vi "Scrap.vi"() -> ()   [LabVIEW 2023]
uses:
  <vilib>/addons/database/Connection.llb/DB Tools Open Connec (String).vi
  <vilib>/regexp/Match Regular Expression.xnode
  <vilib>/addons/database/NI_Database_API.lvlib
panel:
  in  "Quantity":dbl=1.0 min=1.0 max=20.0 step=1.0
  out "DC_SN":string
  in  "Error Code (Electrical)":string(combo)="C30 - Activity Dip"
  in  "Error Code (Electrical +)":string(combo)="C37 - G-Sensitivity"
  in  "Error Code (Post Testing)":string(combo)="C40 - Tinning"
  in  "Work Order":string
  in  "DC_SN":string
  in  "Employee Number":string
  in  "Enter":bool
  in  "Exit":bool
  in  "Comment":string
  in  "Error Code (Pre-Clean Room)":string(combo)="C14 - Dropped"
  in  "Error Code (Post Clean Room)":string(combo)="C38 - Short"
  in  "Location":string(combo)
  in  "Error Code (Clean Room)":string(combo)="C16 - No Oscillate"
  # "Scrapping"
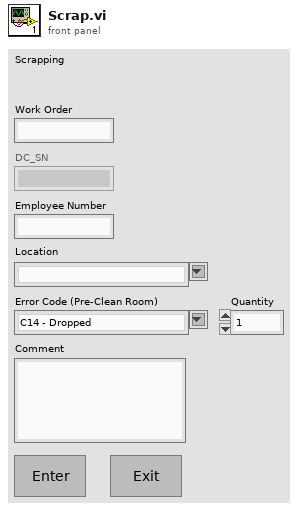
[diagram p1: front panel]
types:
  T1 = typedef "NI_Database_API.lvlib/Conn ObjectReference.ctl" = refnum<k1>
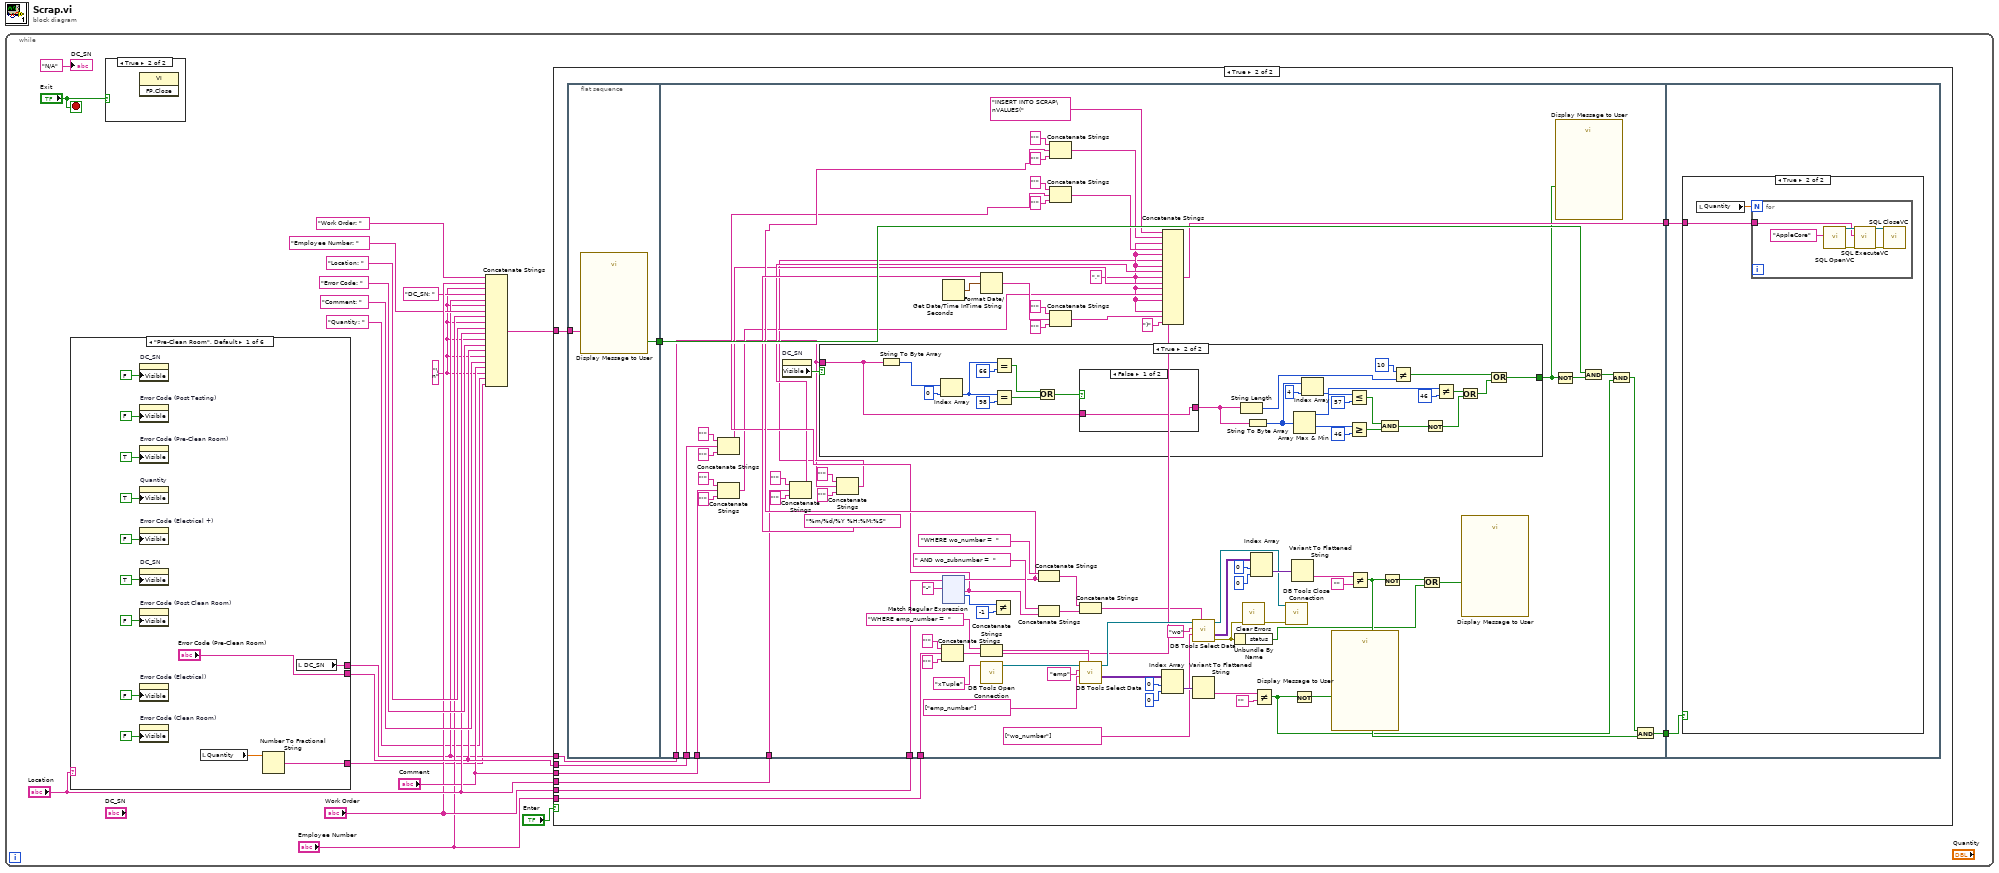
[diagram p0: block diagram]
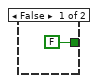
[diagram p4: hidden frame]
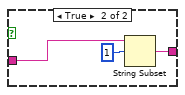
[diagram p5: hidden frame]
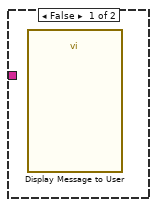
[diagram p6: hidden frame]
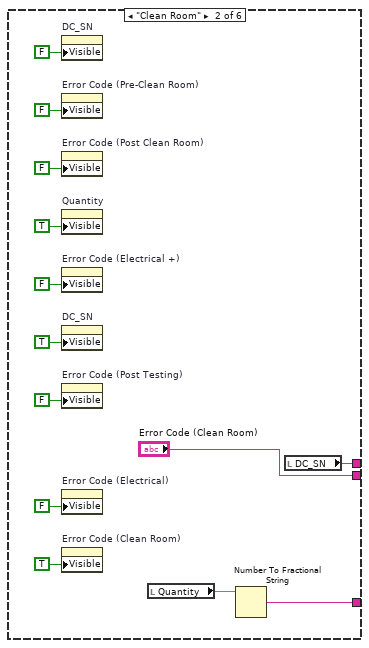
[diagram p7: hidden frame]
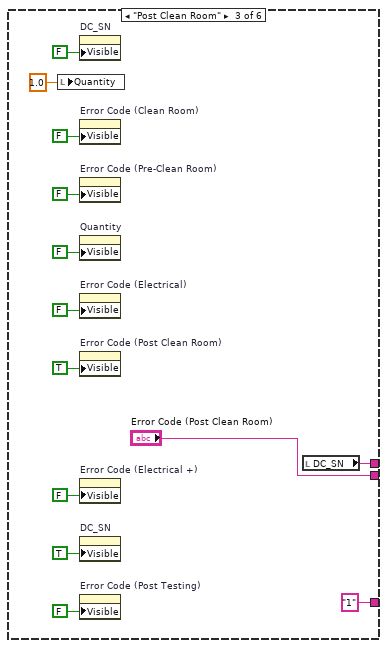
[diagram p8: hidden frame]
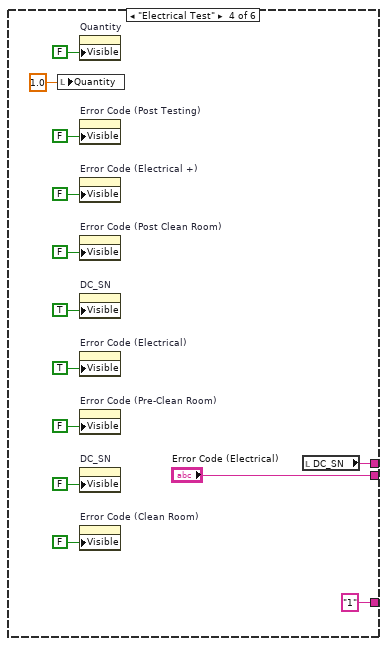
[diagram p9: hidden frame]
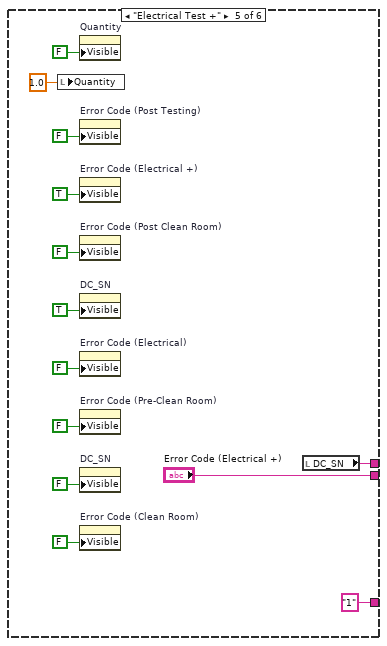
[diagram p10: hidden frame]
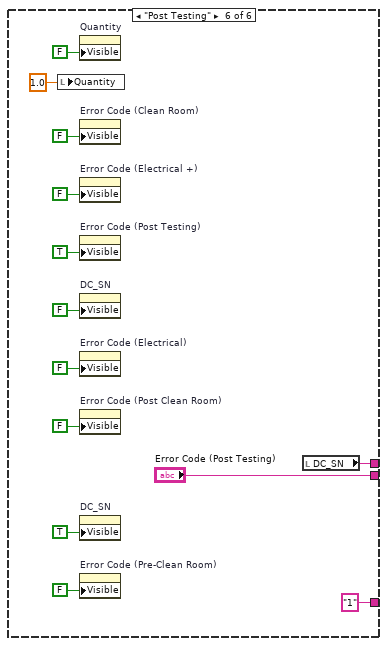
[diagram p11: hidden frame]
diagram:
  n1 = while {
    stop <- "Exit" stop-if-true
    w3 = "\n" ("string")
    n2 = case shown="\"Pre-Clean Room\", Default" "Location" {
      tunnel: ["Error Code (Pre-Clean Room)" "Error Code (Clean Room)" "Error Code (Post Clean Room)" "Error Code (Electrical)" "Error Code (Electrical +)" "Error Code (Post Testing)"] -> w13
      tunnel: [w279 w292 w305 w320 w333 w344] -> w6
      tunnel: [w276 w289 "1" "1" "1" "1"] -> w1
      frame "Pre-Clean Room", Default {
        n3 = property on="DC_SN" class="Str"("Visible"=FALSE) -> ()  [unwired: 2 in, 2 out]
        n4 = property on="Error Code (Post Testing)" class="CmbBox"("Visible"=FALSE) -> ()  [unwired: 2 in, 2 out]
        n5 = property on="Error Code (Pre-Clean Room)" class="CmbBox"("Visible"=TRUE) -> ()  [unwired: 2 in, 2 out]
        n6 = property on="Quantity" class="DigNum (strict)"("Visible"=TRUE) -> ()  [unwired: 2 in, 2 out]
        n7 = property on="Error Code (Electrical +)" class="CmbBox"("Visible"=FALSE) -> ()  [unwired: 2 in, 2 out]
        n8 = property on="DC_SN" class="Str"("Visible"=TRUE) -> ()  [unwired: 2 in, 2 out]
        n9 = property on="Error Code (Post Clean Room)" class="CmbBox"("Visible"=FALSE) -> ()  [unwired: 2 in, 2 out]
        n10 = property on="Error Code (Electrical)" class="CmbBox"("Visible"=FALSE) -> ()  [unwired: 2 in, 2 out]
        n11 = property on="Error Code (Clean Room)" class="CmbBox"("Visible"=FALSE) -> ()  [unwired: 2 in, 2 out]
        n12 = local read "Quantity"() -> (w277:dbl)
        n13 = Number To Fractional String(number=w277) -> (F-format string=w276:string)  [unwired: 3 in]
        n14 = local read "DC_SN"() -> (w279:string)
      }
      frame "Clean Room" {
        n15 = property on="DC_SN" class="Str"("Visible"=FALSE) -> ()  [unwired: 2 in, 2 out]
        n16 = property on="Error Code (Pre-Clean Room)" class="CmbBox"("Visible"=FALSE) -> ()  [unwired: 2 in, 2 out]
        n17 = property on="Error Code (Post Clean Room)" class="CmbBox"("Visible"=FALSE) -> ()  [unwired: 2 in, 2 out]
        n18 = property on="Quantity" class="DigNum (strict)"("Visible"=TRUE) -> ()  [unwired: 2 in, 2 out]
        n19 = property on="Error Code (Electrical +)" class="CmbBox"("Visible"=FALSE) -> ()  [unwired: 2 in, 2 out]
        n20 = property on="DC_SN" class="Str"("Visible"=TRUE) -> ()  [unwired: 2 in, 2 out]
        n21 = property on="Error Code (Post Testing)" class="CmbBox"("Visible"=FALSE) -> ()  [unwired: 2 in, 2 out]
        n22 = property on="Error Code (Electrical)" class="CmbBox"("Visible"=FALSE) -> ()  [unwired: 2 in, 2 out]
        n23 = property on="Error Code (Clean Room)" class="CmbBox"("Visible"=TRUE) -> ()  [unwired: 2 in, 2 out]
        n24 = local read "Quantity"() -> (w290:dbl)
        n25 = Number To Fractional String(number=w290) -> (F-format string=w289:string)  [unwired: 3 in]
        n26 = local read "DC_SN"() -> (w292:string)
      }
      frame "Post Clean Room" {
        n27 = local write "Quantity"(1.0 ("Quantity")) -> ()
        n28 = property on="DC_SN" class="Str"("Visible"=FALSE) -> ()  [unwired: 2 in, 2 out]
        n29 = property on="Error Code (Clean Room)" class="CmbBox"("Visible"=FALSE) -> ()  [unwired: 2 in, 2 out]
        n30 = property on="Error Code (Pre-Clean Room)" class="CmbBox"("Visible"=FALSE) -> ()  [unwired: 2 in, 2 out]
        n31 = property on="Quantity" class="DigNum (strict)"("Visible"=FALSE) -> ()  [unwired: 2 in, 2 out]
        n32 = property on="Error Code (Electrical)" class="CmbBox"("Visible"=FALSE) -> ()  [unwired: 2 in, 2 out]
        n33 = property on="Error Code (Post Clean Room)" class="CmbBox"("Visible"=TRUE) -> ()  [unwired: 2 in, 2 out]
        n34 = property on="Error Code (Electrical +)" class="CmbBox"("Visible"=FALSE) -> ()  [unwired: 2 in, 2 out]
        n35 = property on="DC_SN" class="Str"("Visible"=TRUE) -> ()  [unwired: 2 in, 2 out]
        n36 = property on="Error Code (Post Testing)" class="CmbBox"("Visible"=FALSE) -> ()  [unwired: 2 in, 2 out]
        n37 = local read "DC_SN"() -> (w305:string)
      }
      frame "Electrical Test" {
        n38 = local write "Quantity"(1.0 ("Quantity")) -> ()
        n39 = property on="Quantity" class="DigNum (strict)"("Visible"=FALSE) -> ()  [unwired: 2 in, 2 out]
        n40 = property on="Error Code (Post Testing)" class="CmbBox"("Visible"=FALSE) -> ()  [unwired: 2 in, 2 out]
        n41 = property on="Error Code (Electrical +)" class="CmbBox"("Visible"=FALSE) -> ()  [unwired: 2 in, 2 out]
        n42 = property on="Error Code (Post Clean Room)" class="CmbBox"("Visible"=FALSE) -> ()  [unwired: 2 in, 2 out]
        n43 = property on="DC_SN" class="Str"("Visible"=TRUE) -> ()  [unwired: 2 in, 2 out]
        n44 = property on="Error Code (Electrical)" class="CmbBox"("Visible"=TRUE) -> ()  [unwired: 2 in, 2 out]
        n45 = property on="Error Code (Pre-Clean Room)" class="CmbBox"("Visible"=FALSE) -> ()  [unwired: 2 in, 2 out]
        n46 = property on="DC_SN" class="Str"("Visible"=FALSE) -> ()  [unwired: 2 in, 2 out]
        n47 = property on="Error Code (Clean Room)" class="CmbBox"("Visible"=FALSE) -> ()  [unwired: 2 in, 2 out]
        n48 = local read "DC_SN"() -> (w320:string)
      }
      frame "Electrical Test +" {
        n49 = local write "Quantity"(1.0 ("Quantity")) -> ()
        n50 = property on="Quantity" class="DigNum (strict)"("Visible"=FALSE) -> ()  [unwired: 2 in, 2 out]
        n51 = property on="Error Code (Post Testing)" class="CmbBox"("Visible"=FALSE) -> ()  [unwired: 2 in, 2 out]
        n52 = property on="Error Code (Electrical +)" class="CmbBox"("Visible"=TRUE) -> ()  [unwired: 2 in, 2 out]
        n53 = property on="Error Code (Post Clean Room)" class="CmbBox"("Visible"=FALSE) -> ()  [unwired: 2 in, 2 out]
        n54 = property on="DC_SN" class="Str"("Visible"=TRUE) -> ()  [unwired: 2 in, 2 out]
        n55 = property on="Error Code (Electrical)" class="CmbBox"("Visible"=FALSE) -> ()  [unwired: 2 in, 2 out]
        n56 = property on="Error Code (Pre-Clean Room)" class="CmbBox"("Visible"=FALSE) -> ()  [unwired: 2 in, 2 out]
        n57 = property on="DC_SN" class="Str"("Visible"=FALSE) -> ()  [unwired: 2 in, 2 out]
        n58 = property on="Error Code (Clean Room)" class="CmbBox"("Visible"=FALSE) -> ()  [unwired: 2 in, 2 out]
        n59 = local read "DC_SN"() -> (w333:string)
      }
      frame "Post Testing" {
        n60 = local write "Quantity"(1.0 ("Quantity")) -> ()
        n61 = property on="Quantity" class="DigNum (strict)"("Visible"=FALSE) -> ()  [unwired: 2 in, 2 out]
        n62 = property on="Error Code (Clean Room)" class="CmbBox"("Visible"=FALSE) -> ()  [unwired: 2 in, 2 out]
        n63 = property on="Error Code (Electrical +)" class="CmbBox"("Visible"=FALSE) -> ()  [unwired: 2 in, 2 out]
        n64 = property on="Error Code (Post Testing)" class="CmbBox"("Visible"=TRUE) -> ()  [unwired: 2 in, 2 out]
        n65 = property on="DC_SN" class="Str"("Visible"=FALSE) -> ()  [unwired: 2 in, 2 out]
        n66 = property on="Error Code (Electrical)" class="CmbBox"("Visible"=FALSE) -> ()  [unwired: 2 in, 2 out]
        n67 = property on="Error Code (Post Clean Room)" class="CmbBox"("Visible"=FALSE) -> ()  [unwired: 2 in, 2 out]
        n68 = property on="DC_SN" class="Str"("Visible"=TRUE) -> ()  [unwired: 2 in, 2 out]
        n69 = property on="Error Code (Pre-Clean Room)" class="CmbBox"("Visible"=FALSE) -> ()  [unwired: 2 in, 2 out]
        n70 = local read "DC_SN"() -> (w344:string)
      }
    }
    n71 = case shown="True" "Exit" {
      frame False {
      }
      frame True {
        n72 = invoke class="VI" method="FP.Close"() -> ()  [unwired: 3 in, 3 out]
      }
    }
    n73 = Concatenate Strings("Work Order: " ("string"), "Work Order", w3, "DC_SN: " ("string"), w6, w3, "Employee Number: " ("string"), "Employee Number", w3, "Location: " ("string"), "Location", w3, "Error Code: " ("string"), w13, w3, "Comment: " ("string"), "Comment", w3, "Quantity: " ("string"), w1) -> (w18:string)
    n74 = case shown="True" "Enter" {
      tunnel: w18 -> [_ w29]
      tunnel: "Work Order" -> [_ w26]
      tunnel: "Location" -> [_ w24]
      tunnel: w13 -> [_ w23]
      tunnel: "Comment" -> [_ w22]
      tunnel: "Employee Number" -> [_ w21]
      tunnel: w6 -> [_ w20]
      frame False {
      }
      frame True {
        n75 = flat-sequence {
          tunnel: [w31] -> w28
          tunnel: w29 -> [w30]
          tunnel: w28 -> [w115]
          tunnel: [w33] -> w27
          tunnel: w26 -> [w101]
          tunnel: [w85] -> w25
          tunnel: w24 -> [w71]
          tunnel: w23 -> [w67]
          tunnel: w22 -> [w63]
          tunnel: w21 -> [w59]
          tunnel: w20 -> [w32]
          tunnel: w27 -> [w267]
          tunnel: w25 -> [w266]
          frame #0 {
            n76 = call "Display Message to User"("Message"=w30) -> ("Yes"=w31:bool)  [unwired: 9 in, 1 out]
          }
          frame #1 {
            w49 = "," ("string")
            n77 = Concatenate Strings("'" ("string"), w67, "'" ("string")) -> (w66:string)
            n78 = Concatenate Strings("'" ("string"), w63, "'" ("string")) -> (w62:string)
            n79 = property on="DC_SN" class="Str"() -> ("Visible"=w45:bool)  [unwired: 2 in, 2 out]
            n80 = Concatenate Strings("'" ("string"), w71, "'" ("string")) -> (w70:string)
            n81 = case shown="True" w45 {
              tunnel: w32 -> [_ w121]
              tunnel: [FALSE w127] -> w44
              frame False {
              }
              frame True {
                n82 = String To Byte Array(string=w121) -> (unsigned byte array=w122:u8[])
                n83 = Index Array(array=w122, index=0) -> (element=w120:u8)
                n84 = Equal?(x=w120, y=u8 66) -> (x = y?=w118:bool)
                n85 = Equal?(x=w120, y=u8 98) -> (x = y?=w124:bool)
                n86 = Or(x=w118, y=w124) -> (x .or. y?=w123:bool)
                n87 = case shown="False" w123 {
                  tunnel: w121 -> [w145 w148]
                  tunnel: [w145 w146] -> w117
                  frame False {
                  }
                  frame True {
                    n88 = String Subset(string=w148, offset (0)=1) -> (substring=w146:string)  [unwired: 1 in]
                  }
                }
                n89 = String Length(string=w117) -> (length=w135:i32)
                n90 = String To Byte Array(string=w117) -> (unsigned byte array=w138:u8[])
                n91 = Array Max & Min(array=w138) -> (max value=w140:u8, min value=w139:u8)  [unwired: 2 out]
                n92 = Index Array(array=w138, index=4) -> (element=w136:u8)
                n93 = Less Or Equal?(x=w140, y=u8 57) -> (x <= y?=w141:bool)
                n94 = Greater Or Equal?(x=w139, y=u8 46) -> (x >= y?=w142:bool)
                n95 = And(x=w141, y=w142) -> (x .and. y?=w143:bool)
                n96 = Not Equal?(x=10, y=w135) -> (x != y?=w128:bool)
                n97 = Not(x=w143) -> (.not. x?=w144:bool)
                n98 = Not Equal?(x=w136, y=u8 46) -> (x != y?=w137:bool)
                n99 = Or(x=w137, y=w144) -> (x .or. y?=w129:bool)
                n100 = Or(x=w128, y=w129) -> (x .or. y?=w127:bool)
              }
            }
            n101 = Concatenate Strings("'" ("string"), w32, "'" ("string")) -> (w48:string)
            n102 = Concatenate Strings("'" ("string"), w59, "'" ("string")) -> (w55:string)
            n103 = Get Date/Time In Seconds() -> (seconds since 1Jan1904=w83:timestamp)
            n104 = xnode "Match Regular Expression"("input string"=w101, "regular expression"="-") -> ("before match"=w78:string, "after match"=w76:string, "offset past match"=w47:i32)  [unwired: 4 in, 2 out]
            n105 = Format Date/Time String(time format string (%c)="%m/%d/%Y %H:%M:%S", seconds (now)=w83) -> (date/time string=w84:string)  [unwired: 1 in]
            n106 = Concatenate Strings("WHERE emp_number =  " ("condition"), w55) -> (w105:string)
            n107 = call-poly <vilib>:"DB Tools Open Connection.vi"("connection information"="xTuple" ("Connection Strings")) -> ("connection reference"=w104:T1)  [unwired: 7 in, 1 out]
            n108 = Not Equal?(x=w47, y=-1) -> ()  [unwired: 1 out]
            n109 = Concatenate Strings("WHERE wo_number =  " ("condition"), w78) -> (w41:string)
            n110 = Concatenate Strings(" AND wo_subnumber =  " ("condition"), w76) -> (w42:string)
            n111 = Concatenate Strings("'" ("string"), w78, "'" ("string")) -> (w51:string)
            n112 = Concatenate Strings("'" ("string"), w76, "'" ("string")) -> (w50:string)
            n113 = Concatenate Strings("'" ("string"), w84, "'" ("string")) -> (w58:string)
            n114 = Concatenate Strings(w41, w42) -> (w43:string)
            n115 = call <vilib>:"DB Tools Select Data.vi"("condition"=w105, "columns"=string[] ["emp_number"], "table"="emp", "connection reference"=w104) -> ("data"=w107:variant[][], "connection reference out"=w110:T1)  [unwired: 2 in, 1 out]
            n116 = Index Array(array=w107, index (row)=0, index (col)=0 ("disabled index (col)")) -> (element=w106:variant)
            n117 = Concatenate Strings("INSERT INTO SCRAP\nVALUES(" ("string"), w51, w49, w50, w49, w48, w49, w70, w49, w66, w49, w62, w49, w55, w49, w58, ")" ("string")) -> (w85:string)
            n118 = call <vilib>:"DB Tools Select Data.vi"("condition"=w43, "columns"=string[] ["wo_number"], "table"="wo", "connection reference"=w110) -> ("error out"=w39:errorcluster, "data"=w113:variant[][], "connection reference out"=w40:T1)  [unwired: 2 in]
            n119 = Variant To Flattened String(Variant=w106) -> (data string=w108:string)  [unwired: 1 out]
            n120 = Unbundle By Name(w39) -> ("status"=w36:bool)
            n121 = call <vilib>:"Clear Errors.vi"("error in (no error)"=w39) -> ("error out"=w38:errorcluster)  [unwired: 5 in, 1 out]
            n122 = Index Array(array=w113, index (row)=0, index (col)=0 ("disabled index (col)")) -> (element=w111:variant)
            n123 = Not Equal?(x=w108, y="") -> (x != y?=w34:bool)
            n124 = call <vilib>:"DB Tools Close Connection.vi"("error in (no error)"=w38, "connection reference"=w40) -> ()  [unwired: 5 in, 1 out]
            n125 = Variant To Flattened String(Variant=w111) -> (data string=w112:string)  [unwired: 1 out]
            n126 = Not(x=w34) -> (.not. x?=w109:bool)
            n127 = call "Display Message to User"("Enable"=w109) -> ()  [unwired: 9 in, 2 out]
            n128 = Not Equal?(x=w112, y="") -> (x != y?=w86:bool)
            n129 = Not(x=w86) -> (.not. x?=w37:bool)
            n130 = Or(x=w37, y=w36) -> (x .or. y?=w35:bool)
            n131 = call "Display Message to User"("Enable"=w35) -> ()  [unwired: 9 in, 2 out]
            n132 = Not(x=w44) -> (.not. x?=w114:bool)
            n133 = call "Display Message to User"("Enable"=w44) -> ()  [unwired: 9 in, 2 out]
            n134 = And(x=w115, y=w114) -> (x .and. y?=w88:bool)
            n135 = And(x=w88, y=w34) -> (x .and. y?=w87:bool)
            n136 = And(x=w87, y=w86) -> (x .and. y?=w33:bool)
          }
          frame #2 {
            n137 = case shown="True" w267 {
              tunnel: w266 -> [_ w269]
              frame False {
                n138 = call "Display Message to User"() -> ()  [unwired: 10 in, 2 out]
              }
              frame True {
                n139 = local read "Quantity"() -> (w268:dbl)
                n140 = for {
                  N: w268 -> [_]
                  tunnel: w269 -> [w270]
                  n141 = call "SQL OpenVC.vi"("ConnectionString In"="AppleCore") -> ("Connection Out"=w275:refnum<k7>, "Error out"=w274:errorcluster)  [unwired: 17 in]
                  n142 = call "SQL ExecuteVC.vi"("Connection In"=w275, "SQL Query"=w270, "Error in (no error)"=w274) -> ("Connection Out"=w273:refnum<k7>, "Error out"=w272:errorcluster)  [unwired: 15 in]
                  n143 = call "SQL CloseVC.vi"("Connection In"=w273, "Error in (no error)"=w272) -> ()  [unwired: 17 in, 1 out]
                }
              }
            }
          }
        }
      }
    }
    "DC_SN" <- "N/A" ("DC_SN")
  }
